vi "main.vi"() -> ()   [LabVIEW 2015]
uses:
  <vilib>/Platform/TimedLoop/XDataNode/timing_clust.ctl
  <vilib>/Platform/TimedLoop/XDataNode/nitl_modes.ctl
  <vilib>/Platform/TimedLoop/XDataNode/wakeup.ctl
  <vilib>/platform/TimedLoop/XDataNode/XDataNode.xnode
  <userlib>/SCANalone4x64/SCANalone4x64.lvlib
  <vilib>/Platform/TimedLoop/XDataNode/XDNodeRunTimeDep.lvlib
panel:
  in  "Period":i64
  in  "samplesx":i32=128
  in  "stepx":i16=1
  in  "samplesy":i32=128
  in  "stepy":i16=1
  in  "startx":i16
  in  "starty":i16
  out "Error Out":errorcluster
  in  "Error In":errorcluster
  in  "Correction file path":string="D:/amarcos/Documentos/JRipoll/ScanCube/scancube_jaguirre/gridscancube/Correction Files/Cor_1to1.ctb"
  out "String":string
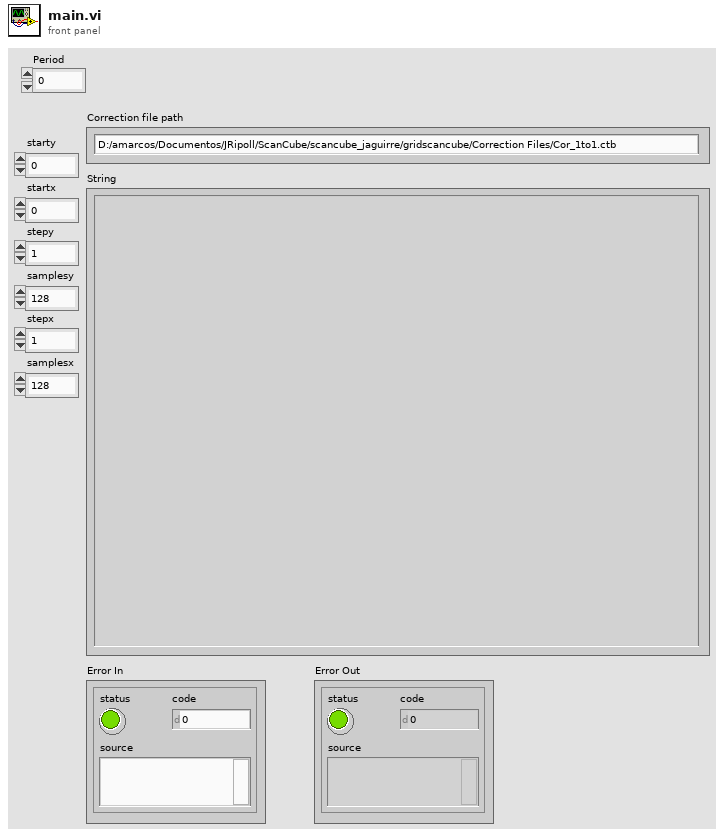
[diagram p1: front panel]
types:
  T1 = typedef "XDNodeRunTimeDep.lvlib/timing_clust.ctl" = cluster{"Expected End [f-1]":u64, "Actual End [f-1]":u64, "Finished Late? [f-1]":bool, "Expected End [i-1]":u64, "Actual End [i-1]":u64, "Finished Late? [i-1]":bool, "Expected Start [i]":u64, "Actual Start [i]":u64, "Expected Start [f]":u64, "Actual Start [f]":u64, "Source Name":string, "Structure Name":string, "Period":i64, "Deadline":i64, "Offset":i64, "Start":i64, "Priority":i32, "Timeout":i32, "Mode":T2, "Wakeup Reason":T3, "Error":errorcluster, "Source Type":string, "Secondary Source Type":string, "Global End Time":u64, "Global Start Time":u64, "Frame Duration":u64, "Iteration Duration":u64, "Assigned CPU":i32, "I/O Scan Engine Mode":u32}
  T2 = typedef "XDNodeRunTimeDep.lvlib/nitl_modes.ctl" = enum32{"No Change", "Process missed periods, maintain original phase", "Discard missed periods, maintain original phase", "Process missed periods, ignore original phase", "Discard missed periods, ignore original phase"}
  T3 = typedef "XDNodeRunTimeDep.lvlib/wakeup.ctl" = enum32{"Normal", "Aborted", "Asynchronous wakeup", "Timing source error", "Timed loop error", "Timeout"}
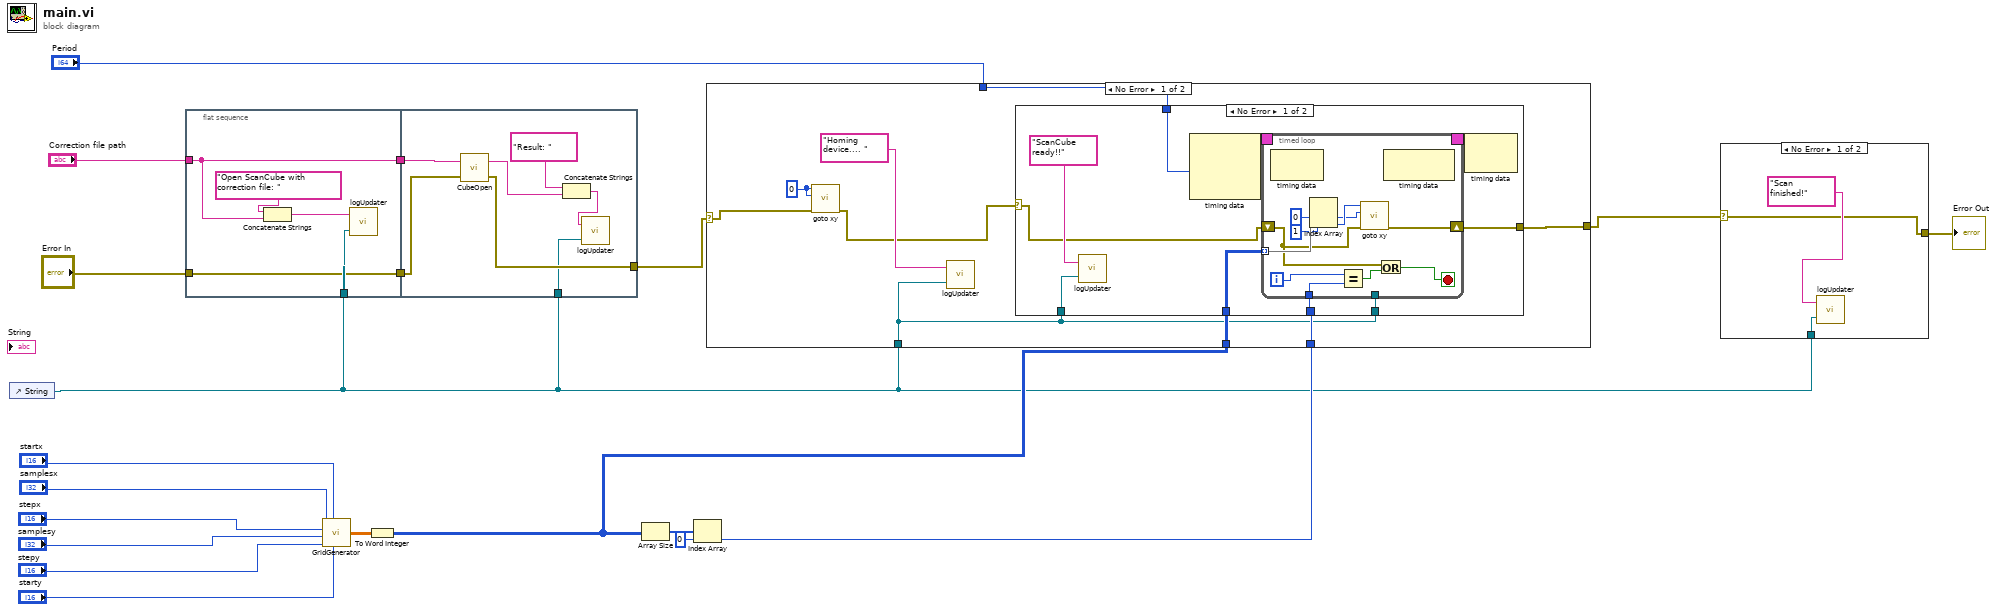
[diagram p0: block diagram]
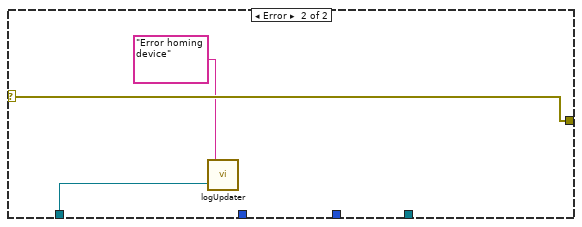
[diagram p3: hidden frame]
diagram:
  n1 = control-ref of="String"() -> (w2:refnum<vi>)
  n2 = flat-sequence {
    tunnel: "Correction file path" -> [w24]
    tunnel: [w24] -> w19
    tunnel: w2 -> [w22]
    tunnel: [w21] -> w18
    tunnel: "Error In" -> [w21]
    tunnel: w19 -> [w32]
    tunnel: w18 -> [w31]
    tunnel: [w30] -> w4
    tunnel: w2 -> [w29]
    frame #0 {
      n3 = Concatenate Strings("Open ScanCube with correction file: ", w24) -> (w23:string)
      n4 = call "logUpdater.vi"("Response"=w22, "Input"=w23) -> ()  [unwired: 1 out]
    }
    frame #1 {
      n5 = call "CubeOpen.vi"("Error In"=w31, "filename"=w32) -> ("Error Out"=w30:errorcluster, "String"=w27:string)
      n6 = Concatenate Strings("Result: ", w27) -> (w26:string)
      n7 = call "logUpdater.vi"("Response"=w29, "Input"=w26) -> ()  [unwired: 1 out]
    }
  }
  n8 = call "GridGenerator.vi"("starty"="starty", "startx"="startx", "stepy"="stepy", "samplesy"="samplesy", "stepx"="stepx", "samplesx"="samplesx") -> ("appended array"=w11:dbl[][])
  n9 = To Word Integer(number=w11) -> (16bit integer=w7:i16[][])
  n10 = Array Size(array=w7) -> (size(s)=w10:i32[])
  n11 = Index Array(array=w10, index=0) -> (element=w8:i32)
  n12 = case shown="No Error" w4 {
    selector: w4 -> [w38 w72]
    tunnel: w8 -> [w37 _]
    tunnel: w7 -> [w41 _]
    tunnel: w2 -> [w33 _]
    tunnel: "Period" -> [w40 _]
    tunnel: [w39 w72] -> w3
    frame No Error {
      w36 = i16 0 ("x")
      n13 = call <userlib>:"goto xy.vi"("error in (no error)"=w38, "y"=w36, "x"=w36) -> ("error out"=w34:errorcluster)  [unwired: 8 in]
      n14 = call "logUpdater.vi"("Response"=w33, "Input"="Homing device.... ") -> ()  [unwired: 1 out]
      n15 = case shown="No Error" w34 {
        selector: w34 -> [w42 w71]
        tunnel: w41 -> [w49 _]
        tunnel: w40 -> [w48 _]
        tunnel: [w47 w71] -> w39
        tunnel: w33 -> [w46 _]
        tunnel: w37 -> [w45 _]
        tunnel: w33 -> [w44 w70]
        frame No Error {
          n16 = call "logUpdater.vi"("Response"=w44, "Input"="ScanCube ready!!") -> ()  [unwired: 1 out]
          n17 = node-c288(w48) -> (w51:T1)  [unwired: 2 in]
          n18 = timed-loop {
            tunnel: w46 -> [_]
            tunnel: w49 -> [w62] mode=indexing
            timing: w51 -> [_]
            timing-out: [_] -> w50
            tunnel: w45 -> [w58]
            shift-right: [w54] -> w47
            shift-left: w42 -> [w52]
            i -> [w59]
            stop <- w55 stop-if-true
            n19 = node-c288() -> ()  [unwired: 1 in, 1 out]
            n20 = Index Array(array=w62, index #1=0 ("index"), index #2=1 ("index")) -> (element #1=w56:i16, element #2=w57:i16)
            n21 = Equal?(x=w59, y=w58) -> (x = y?=w53:bool)
            n22 = call <userlib>:"goto xy.vi"("error in (no error)"=w52, "y"=w56, "x"=w57) -> ("error out"=w54:errorcluster)  [unwired: 8 in]
            n23 = Or(x=w52, y=w53) -> (x .or. y?=w55:bool)
            n24 = node-c288() -> ()  [unwired: 1 in, 1 out]
          }
          n25 = node-c288(w50) -> ()  [unwired: 1 out]
        }
        frame Error {
          n26 = call "logUpdater.vi"("Response"=w70, "Input"="Error homing device") -> ()  [unwired: 1 out]
        }
      }
    }
    frame Error {
    }
  }
  n27 = case shown="No Error" w3 {
    selector: w3 -> [w73 w76]
    tunnel: w2 -> [w74 _]
    tunnel: [w73 w76] -> w1
    frame No Error {
      n28 = call "logUpdater.vi"("Response"=w74, "Input"="Scan finished!") -> ()  [unwired: 1 out]
    }
    frame Error {
    }
  }
  "Error Out" <- w1
